vi "Is Set.vi"(8 "error in (no error)":errorcluster, 11 "packed in":refnum<class "packed.lvclass">) -> (0 "error out":errorcluster, 2 "Is Set":bool, 3 "packed out":refnum<class "packed.lvclass">)   [LabVIEW 2020, in "Protobuf RAW.lvlib" / "packed.lvclass"]
uses:
  packed.lvclass
  packed.lvclass/packed.ctl
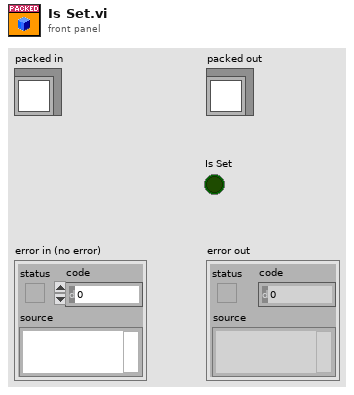
[diagram p1: front panel]
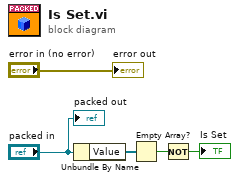
[diagram p0: block diagram]
diagram:
  n1 = Unbundle By Name("packed in") -> ("Value"=w4:refnum<class "Scalar Type.lvclass">[])
  n2 = Empty Array?(array=w4) -> (empty?=w3:bool)
  n3 = Not(x=w3) -> (.not. x?=→"Is Set":bool)
  "error out" <- "error in (no error)"
  "packed out" <- "packed in"
